vi "SLSC Create Bank Properties.vi"(9 "RevA?":bool, 11 "Bank Number":i32) -> (2 "Bank Number Channel":string, 3 "Outgoing configuration":T1[](array[typedef])=[{"Channel Name"="", "SLSC Name"="", "Configuration"={"Type"=enum."Input", "Units"="", "Default Value"=0.0, "Faultable"=FALSE, "Scalable"=FALSE}, "Enum Names"=[], "Enum Values"=[]}, {"Channel Name"="", "SLSC Name"="", "Configuration"={"Type"=enum."Input", "Units"="", "Default Value"=0.0, "Faultable"=FALSE, "Scalable"=FALSE}, "Enum Names"=[], "Enum Values"=[]}])   [LabVIEW 2015, in "SLSC-12201 DIO System Explorer.lvlib"]
uses:
  SLSC-12201 DIO System Explorer.lvlib
  Shared/SLSC Channel Information.ctl
  <vilib>/NI Veristand/Custom Device API/Custom Device Channel.ctl
  <vilib>/NI Veristand/Custom Device API/Custom Device Channel Type.ctl
  <vilib>/NI Veristand/Custom Device API/Custom Device API.lvlib
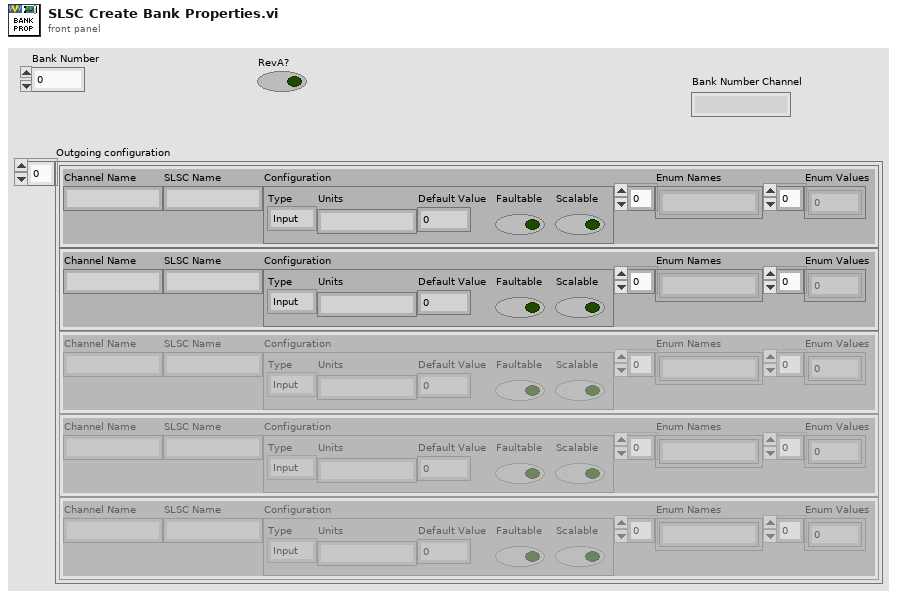
[diagram p1: front panel]
types:
  T1 = typedef "SLSC-12201 DIO System Explorer.lvlib/SLSC Channel Information.ctl" = cluster{"Channel Name":string, "SLSC Name":string, "Configuration":T2, "Enum Names":string[], "Enum Values":i32[]}
  T2 = typedef "Custom Device API.lvlib/Custom Device Channel.ctl" = cluster{"Type":T3, "Units":string, "Default Value":dbl, "Faultable":bool, "Scalable":bool}
  T3 = typedef "Custom Device API.lvlib/Custom Device Channel Type.ctl" = enum16{"Input", "Output"}
  T4 = cluster{"Channel Name":string, "SLSC Name":string, "Enum Names":string[], "Enum Values":i32[]}
  T5 = cluster{"Channel Name":string, "SLSC Name":string, "Enum Names":string[], "Enum Values":i32[]}[]
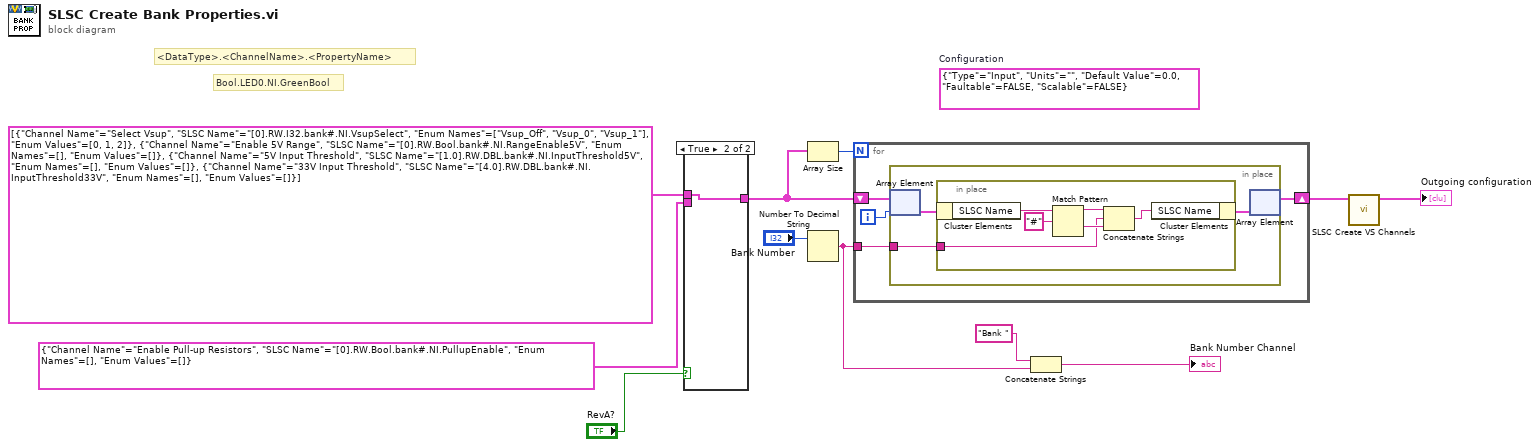
[diagram p0: block diagram]
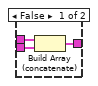
[diagram p2: hidden frame]
diagram:
  (unwired) T2 {"Type"=enum."Input", "Units"="", "Default Value"=0.0, "Faultable"=FALSE, "Scalable"=FALSE}  # Configuration
  # "Bool.LED0.NI.GreenBool"
  # "<DataType>.<ChannelName>.<PropertyName>"
  n1 = case shown="True" "RevA?" {
    tunnel: T5 [{"Channel Name"="Select Vsup", "SLSC Name"="[0].RW.I32.bank#.NI.VsupSelect", "Enum Names"=["Vsup_Off", "Vsup_0", "Vsup_1"], "Enum Values"=[0, 1, 2]}, {"Channel Name"="Enable 5V Range", "SLSC Name"="[0].RW.Bool.bank#.NI.RangeEnable5V", "Enum Names"=[], "Enum Values"=[]}, {"Channel Name"="5V Input Threshold", "SLSC Name"="[1.0].RW.DBL.bank#.NI.InputThreshold5V", "Enum Names"=[], "Enum Values"=[]}, {"Channel Name"="33V Input Threshold", "SLSC Name"="[4.0].RW.DBL.bank#.NI.InputThreshold33V", "Enum Names"=[], "Enum Values"=[]}] -> [w14 w15]
    tunnel: [w13 w15] -> w8
    tunnel: T4 {"Channel Name"="Enable Pull-up Resistors", "SLSC Name"="[0].RW.Bool.bank#.NI.PullupEnable", "Enum Names"=[], "Enum Values"=[]} -> [w12 _]
    frame False {
      n2 = Build Array (concatenate)(w14, w12) -> (w13:T5)
    }
    frame True {
    }
  }
  n3 = Array Size(array=w8) -> (size(s)=w11:i32)
  n4 = Number To Decimal String(number="Bank Number") -> (decimal integer string=w2:string)  [unwired: 1 in]
  n5 = for {
    N: w11 -> [_]
    shift-right: [w18] -> w6
    shift-left: w8 -> [w19]
    tunnel: w2 -> [w16]
    i -> [w17]
    n6 = in-place {
      in-place-border: w16 -> [w20]
      n7 = in-place-array #1(w19, w17) -> (w22:T4)
      n8 = in-place {
        in-place-border: w20 -> [w24]
        n9 = in-place-cluster #2(w22) -> ("SLSC Name"=w28:string)
        n10 = Match Pattern(string=w28, regular expression="#") -> (before substring=w26:string, after substring=w25:string)  [unwired: 1 in, 2 out]
        n11 = Concatenate Strings(w26, w24, w25) -> (w23:string)
        n12 = in-place-cluster #2("SLSC Name"=w23) -> (w21:T4)
      }
      n13 = in-place-array #1(w21) -> (w18:T5)  [unwired: 1 out]
    }
  }
  n14 = Concatenate Strings("Bank " ("string"), w2) -> (→"Bank Number Channel":string)
  n15 = call "SLSC Create VS Channels.vi"("Array in"=w6) -> ("Array out"=→"Outgoing configuration":T1[])  [unwired: 10 in]
